vi "Set f0.vi"(8 "error in":errorcluster, 10 "f0":sgl, 11 "PAS Data in":refnum<class "PAS Data.lvclass">) -> (0 "error out":errorcluster, 3 "PAS Data out":refnum<class "PAS Data.lvclass">)   [LabVIEW 2015, in "PAS Data.lvclass"]
uses:
  PAS Data.lvclass
  PAS Data.lvclass/PAS Data.ctl
  Cell/PAS Cell Data.lvclass
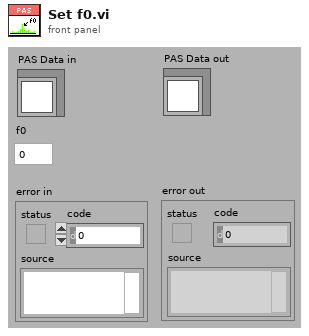
[diagram p1: front panel]
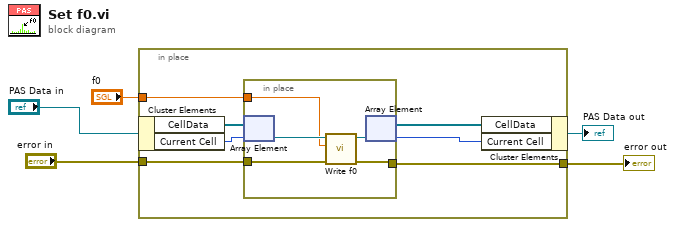
[diagram p0: block diagram]
diagram:
  n1 = in-place {
    in-place-border: "f0" -> [w10]
    in-place-border: "error in" -> [w7]
    in-place-border: [w6] -> w2
    n2 = in-place-cluster #1("PAS Data in") -> ("CellData"=w12:refnum<class "PAS Cell Data.lvclass">[], "Current Cell"=w11:i32)
    n3 = in-place {
      in-place-border: w10 -> [w16]
      in-place-border: w7 -> [w14]
      in-place-border: [w13] -> w6
      n4 = in-place-array #2(w12, w11) -> (w17:refnum<class "PAS Cell Data.lvclass">)
      n5 = call "Write f0.vi"("error in (no error)"=w14, "f0"=w16, "PAS Cell Data in"=w17) -> ("error out"=w13:errorcluster, "PAS Cell Data out"=w15:refnum<class "PAS Cell Data.lvclass">)  [unwired: 7 in]
      n6 = in-place-array #2(w15) -> (w9:refnum<class "PAS Cell Data.lvclass">[], w8:i32)
    }
    n7 = in-place-cluster #1("CellData"=w9, "Current Cell"=w8) -> (→"PAS Data out":refnum<class "PAS Data.lvclass">)
  }
  "error out" <- w2
